vi "S2DS_ConfigReadRC (SubVI).vi"(0 "Refnum in":T3, 1 "RC Info list (in)":T1, 3 "error in (no error)":errorcluster) -> (6 "Refnum out":T3, 7 "RC Info list (out)":T1, 9 "error out":errorcluster)   [LabVIEW 2016]
uses:
  <vilib>/Utility/config.llb/Config Data RefNum.ctl
  TYPE DEFS/S2DS_RC info.ctl
  TYPE DEFS/S2DS_Single RC info.ctl
  <vilib>/Utility/config.llb/Read Key (U32).vi
  <vilib>/Utility/config.llb/Read Key (String).vi
  <vilib>/Utility/config.llb/Read Key (Double).vi
  <vilib>/Utility/config.llb/NI_LVConfig.lvlib
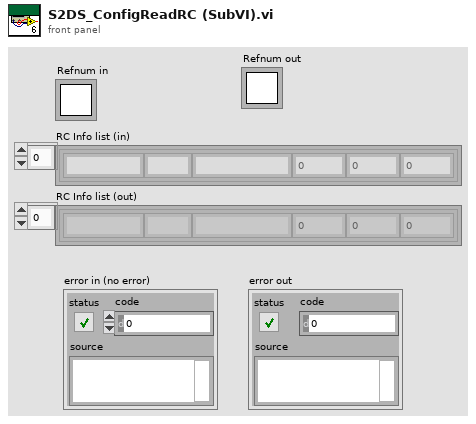
[diagram p1: front panel]
types:
  T1 = typedef "S2DS_RC info.ctl" = T2[]
  T2 = typedef "S2DS_Single RC info.ctl" = cluster{"Instrument identifier":string, "Factor":dbl, "Averaging":i32, "Wait (ms)":i32, "Unit":string, "Name":string}
  T3 = typedef "NI_LVConfig.lvlib/Config Data RefNum.ctl" = refnum<k1>
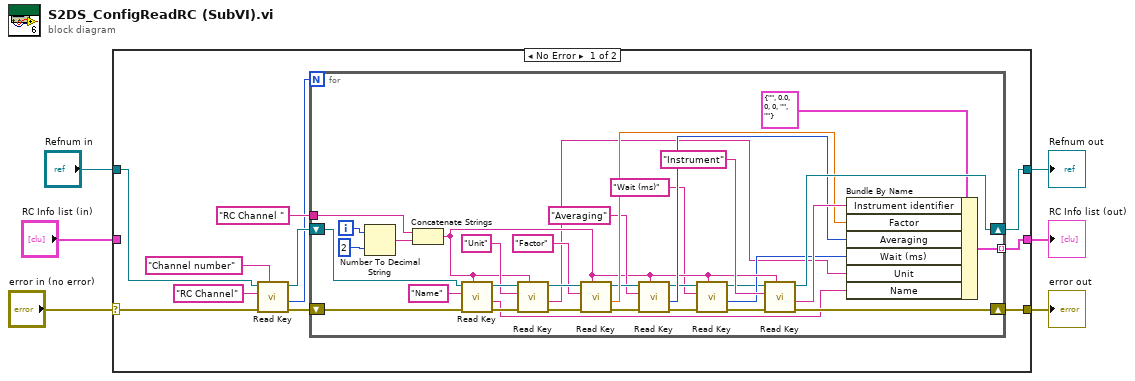
[diagram p0: block diagram]
diagram:
  n1 = case shown="No Error" "error in (no error)" {
    selector: "error in (no error)" -> [w7 w52]
    tunnel: [w17 w52] -> w6
    tunnel: [w16 w51] -> w5
    tunnel: [w15 w53] -> w4
    tunnel: "Refnum in" -> [w11 w51]
    tunnel: "RC Info list (in)" -> [_ w53]
    frame No Error {
      n2 = call-poly <vilib>:"Read Key.vi"("section"="Channel number", "error in (no error)"=w7, "key"="RC Channel", "refnum"=w11) -> ("error out"=w9:errorcluster, "value"=w8:u32, "refnum out"=w10:T3)  [unwired: 1 in, 4 out]
      n3 = for {
        N: w8 -> [_]
        shift-right: [w35] -> w16
        shift-left: w10 -> [w50]
        shift-right: [w34] -> w17
        shift-left: w9 -> [w49]
        tunnel: "RC Channel " -> [w45]
        tunnel: [w38] -> w15 mode=indexing
        i -> [w46]
        n4 = Number To Decimal String(number=w46, width (-)=i16 2) -> (decimal integer string=w48:string)
        n5 = Concatenate Strings(w45, w48) -> (w25:string)
        n6 = call-poly <vilib>:"Read Key.vi"("section"=w25, "error in (no error)"=w49, "key"="Name", "refnum"=w50) -> ("error out"=w42:errorcluster, "value"=w18:string, "refnum out"=w43:T3)  [unwired: 2 in, 3 out]
        n7 = call-poly <vilib>:"Read Key.vi"("section"=w25, "error in (no error)"=w42, "key"="Unit", "refnum"=w43) -> ("error out"=w40:errorcluster, "value"=w19:string, "refnum out"=w39:T3)  [unwired: 2 in, 3 out]
        n8 = call-poly <vilib>:"Read Key.vi"("section"=w25, "error in (no error)"=w40, "key"="Factor", "refnum"=w39) -> ("error out"=w30:errorcluster, "value"=w32:dbl, "refnum out"=w31:T3)  [unwired: 1 in, 4 out]
        n9 = call-poly <vilib>:"Read Key.vi"("section"=w25, "error in (no error)"=w30, "key"="Averaging", "refnum"=w31) -> ("error out"=w26:errorcluster, "value"=w28:u32, "refnum out"=w27:T3)  [unwired: 1 in, 4 out]
        n10 = call-poly <vilib>:"Read Key.vi"("section"=w25, "error in (no error)"=w26, "key"="Wait (ms)", "refnum"=w27) -> ("error out"=w21:errorcluster, "value"=w23:u32, "refnum out"=w22:T3)  [unwired: 1 in, 4 out]
        n11 = call-poly <vilib>:"Read Key.vi"("section"=w25, "error in (no error)"=w21, "key"="Instrument", "refnum"=w22) -> ("error out"=w34:errorcluster, "value"=w36:string, "refnum out"=w35:T3)  [unwired: 2 in, 3 out]
        n12 = Bundle By Name(cluster=T2 {"Instrument identifier"="", "Factor"=0.0, "Averaging"=0, "Wait (ms)"=0, "Unit"="", "Name"=""} ("Write channel info"), "Instrument identifier"=w36, "Factor"=w32, "Averaging"=w28, "Wait (ms)"=w23, "Unit"=w19, "Name"=w18) -> (w38:T2)
      }
    }
    frame Error {
    }
  }
  "error out" <- w6
  "Refnum out" <- w5
  "RC Info list (out)" <- w4
